vi "Find Peak Attributes.vi"(0 "Intensity Data":dbl[](array[numeric]), 1 "Peak Threshold":dbl format="%0.2f", 2 "Pixel Saturation":dbl=225.0, 3 "error in (no error)":errorcluster) -> (4 "Half Width XY Plot":cluster{dbl[], dbl[]}, 5 "peak location":dbl, 6 "peak amplitude":dbl, 7 "peak width":dbl, 8 "error out":errorcluster)   [LabVIEW 2012]
uses:
  <vilib>/Analysis/NI_AAL_SigProc.lvlib
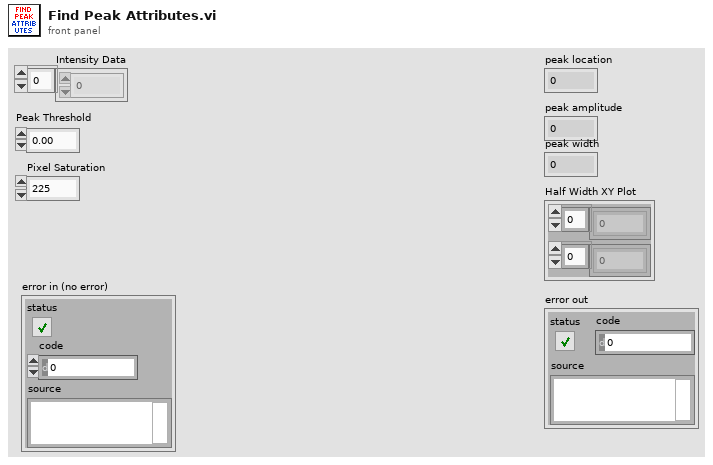
[diagram p1: front panel]
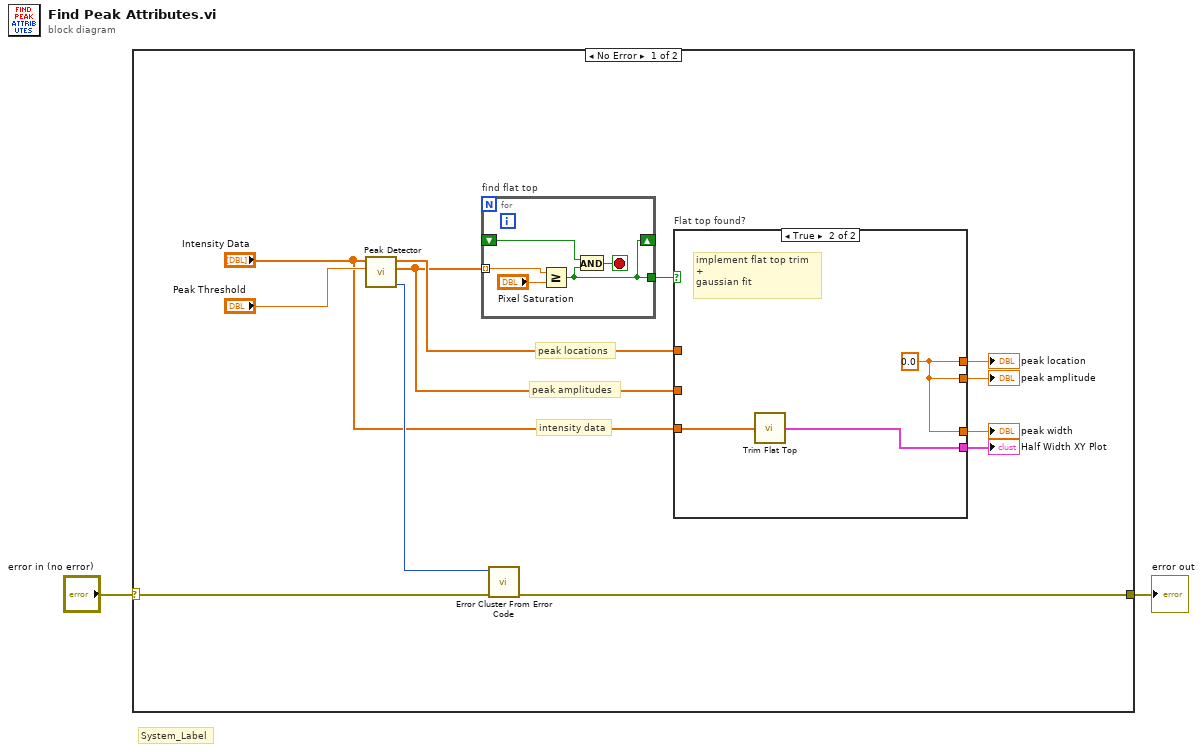
[diagram p0: block diagram]
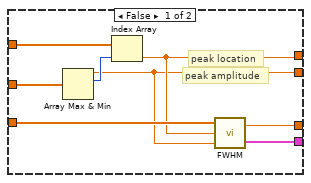
[diagram p2: hidden frame]
diagram:
  # "System_Label"
  n1 = case shown="No Error" "error in (no error)" {
    selector: "error in (no error)" -> [w8 w31]
    tunnel: [w4 w31] -> w1
    frame No Error {
      # "intensity data"
      # "peak amplitudes"
      # "peak locations"
      n2 = call <vilib>:"Peak Detector.vi"("threshold"="Peak Threshold", "X"="Intensity Data") -> ("error"=w13:i32, "Amplitudes"=w10:dbl[], "Locations"=w11:dbl[])  [unwired: 5 in, 2 out]
      n3 = for "find flat top" {
        tunnel: w10 -> [w29] mode=indexing
        tunnel: [w26] -> w12
        shift-right: [w26] -> _
        shift-left: _ -> [w27]
        stop <- w28 stop-if-true
        n4 = Greater Or Equal?(x=w29, y="Pixel Saturation") -> (x >= y?=w26:bool)
        n5 = And(x=w27, y=w26) -> (x .and. y?=w28:bool)
      }
      n6 = call <vilib>:"Error Cluster From Error Code.vi"("error in (no error)"=w8, "error code (0)"=w13) -> ("error out"=w4:errorcluster)  [unwired: 7 in]
      n7 = case "Flat top found?" shown="True" w12 {
        tunnel: w11 -> [w20 _]
        tunnel: w10 -> [w22 _]
        tunnel: [w17 w23] -> w6
        tunnel: [w18 w23] -> w7
        tunnel: "Intensity Data" -> [w19 w25]
        tunnel: [w16 w23] -> w5
        tunnel: [w15 w24] -> w3
        frame False {
          # "peak amplitude"
          # "peak location"
          n8 = Array Max & Min(array=w22) -> (max value=w17:dbl, max index (indices)=w21:i32)  [unwired: 2 out]
          n9 = Index Array(array=w20, index=w21) -> (element=w18:dbl)
          n10 = call "FWHM.vi"("Peak Amplitude"=w17, "Peak Location"=w18, "Intensity Data"=w19) -> ("Half Width XY Plot"=w15:cluster{dbl[], dbl[]}, "Width"=w16:dbl)
        }
        frame True {
          w23 = 0.0
          # "implement flat top trim\n+\ngaussian fit"
          n11 = call "Trim Flat Top.vi"("Intensity Data"=w25) -> ("Data Out (x,y)"=w24:cluster{i32[], dbl[]})
        }
      }
      "peak location" <- w7
      "peak amplitude" <- w6
      "peak width" <- w5
      "Half Width XY Plot" <- w3
    }
    frame Error {
    }
  }
  "error out" <- w1
